vi "Fetch gRPC from Map.vi"(7 "gRPC Server Class type":refnum<class "ServiceBase.lvclass">, 8 "error in (no error)":errorcluster, 11 "Plugin Manager in":refnum<class "CIFPluginManager.lvclass">) -> (0 "error out":errorcluster, 2 "gRPC Server Class out":refnum<class "ServiceBase.lvclass">, 3 "Plugin Manager out":refnum<class "CIFPluginManager.lvclass">)   [LabVIEW 2021, in "CIFPluginManager.lvclass"]
uses:
  CIFPluginManager.lvclass
  <vilib>/gRPC/LabVIEW gRPC Servicer/ServiceBase/ServiceBase.lvclass
  CIFCore/Common/Typedef/Errors.ctl
  CIFPluginManager.lvclass/CIFPluginManager.ctl
  CIFCore/Common/Utilities/Append Error Location.vi
  CIFCore/Common/CIFCoreCommon.lvlib
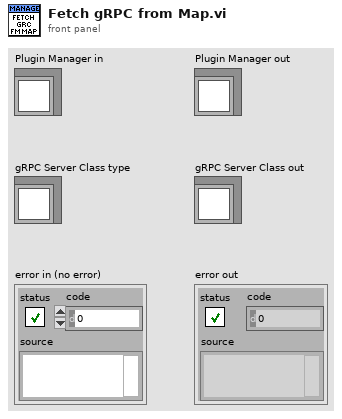
[diagram p1: front panel]
types:
  T1 = typedef "CIFCoreCommon.lvlib/Errors.ctl" = enum16{"Invalid Clock ID", "Long Sleep", "gRPC Server Not Found", "Config Parse", "Timestamp Wrap", "Delayed Execution", "Duplicate Channel", "Missing Channel", "Incorrect Type", "Flatten Error", "Unflatten Data", "Unique Name", "Plugin Not Found"}
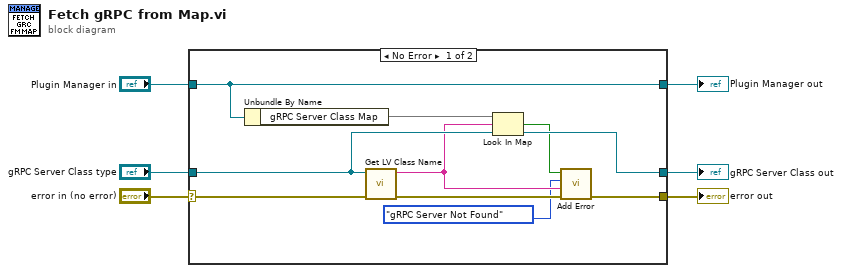
[diagram p0: block diagram]
diagram:
  n1 = case shown="No Error" "error in (no error)" {
    selector: "error in (no error)" -> [w15 w18]
    tunnel: [w10 w18] -> w1
    tunnel: [w16 w19] -> w3
    tunnel: "Plugin Manager in" -> [w16 w19]
    tunnel: "gRPC Server Class type" -> [w12 w17]
    tunnel: [w13 w17] -> w6
    frame No Error {
      n2 = Unbundle By Name(w16) -> ("gRPC Server Class Map"=w14:map{string, refnum<class "ServiceBase.lvclass">})
      n3 = call <vilib>:"Get LV Class Name.vi"("error in (no error)"=w15, "object"=w12) -> ("error out"=w11:errorcluster, "class name"=w9:string)  [unwired: 8 in]
      n4 = Look In Map(map=w14, key=w9, default value=w12) -> (key not found?=w8:bool, value=w13:refnum<class "ServiceBase.lvclass">)
      n5 = call "Add Error.vi"("error in (no error)"=w11, "String to Append"=w9, "Error"=Errors."gRPC Server Not Found", "Insert Error"=w8) -> ("error out"=w10:errorcluster)  [unwired: 7 in]
    }
    frame Error {
    }
  }
  "error out" <- w1
  "Plugin Manager out" <- w3
  "gRPC Server Class out" <- w6
